vi "2039_hw InitDTTalons.vi"(6 "Brake / Coast Mode":T6, 7 "Ramp Rate (Percent/s)":dbl, 8 "error in (no error)":errorcluster, 10 "Enable VComp":bool, 11 "DT Talon Ref Array":T1[](array[typedef])) -> (0 "error out":errorcluster, 3 "DT Talon Ref Array":T1[](array[typedef]))   [LabVIEW 2016, in "2039lib.lvlib"]
uses:
  2039lib.lvlib
  <vilib>/Rock Robotics/WPI/MotorControl/WPI_MotorControlDeviceRef.ctl
  <vilib>/Rock Robotics/WPI/MotorControl/WPI_MotorControlType.ctl
  <vilib>/Rock Robotics/SystemInterfaces/DIO/FPGA_DIOPWMChannel.ctl
  <vilib>/Rock Robotics/WPI/PWM/WPI_PWMDeadband.ctl
  <vilib>/Rock Robotics/WPI/ThirdParty/CanMotor/TalonSRX/WPI_CANTalonSRX_BrakeOverride.ctl
  <vilib>/Rock Robotics/WPI/ThirdParty/CanMotor/TalonSRX/WPI_CANTalonSRX_APIFeedbackSelect.ctl
  <vilib>/Rock Robotics/WPI/ThirdParty/CanMotor/TalonSRX/WPI_CANTalonSRX_APIControlMode.ctl
panel:
  in  "Feedback Reference":T5
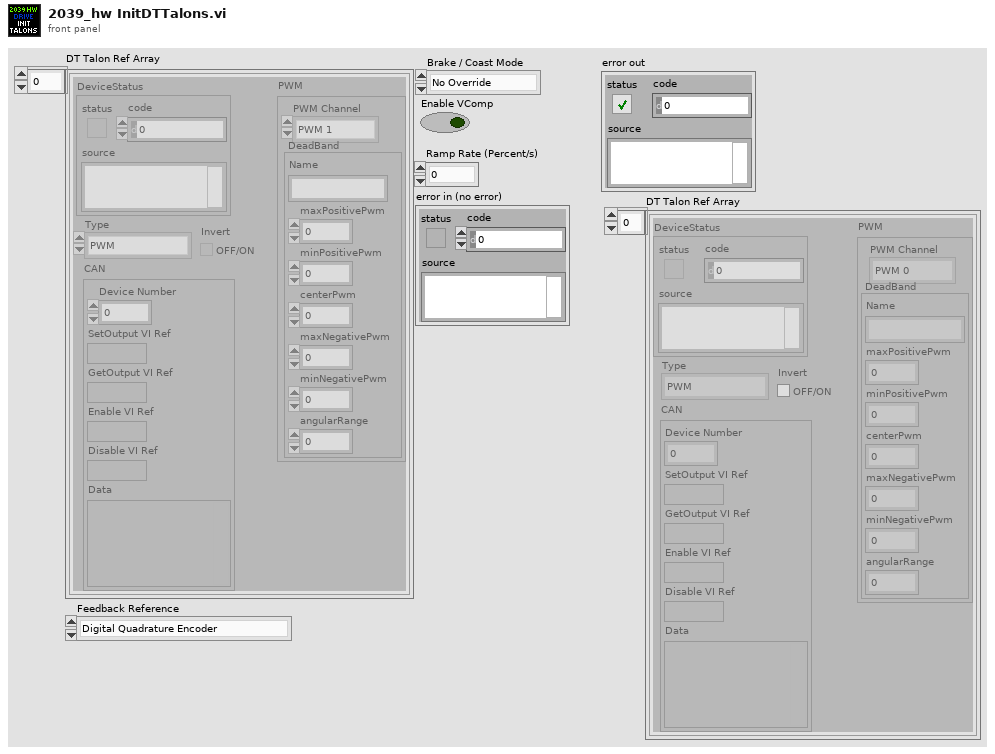
[diagram p1: front panel]
types:
  T1 = typedef "WPI_MotorControlDeviceRef.ctl" = cluster{"DeviceStatus":errorcluster, "Type":T2, "PWM":cluster{"PWM Channel":T3, "DeadBand":T4}, "CAN":cluster{"Device Number":u8, "SetOutput VI Ref":variant, "GetOutput VI Ref":variant, "Enable VI Ref":variant, "Disable VI Ref":variant, "Data":variant}, "Invert":bool}
  T2 = typedef "WPI_MotorControlType.ctl" = enum16{"PWM", "CAN"}
  T3 = typedef "FPGA_DIOPWMChannel.ctl" = enum8{"PWM 0", "PWM 1", "PWM 2", "PWM 3", "PWM 4", "PWM 5", "PWM 6", "PWM 7", "PWM 8", "PWM 9", "PWM MXP 0", "PWM MXP 1", "PWM MXP 2", "PWM MXP 3", "PWM MXP 4", "PWM MXP 5", "PWM MXP 6", "PWM MXP 7", "PWM MXP 8", "PWM MXP 9", "Invalid"}
  T4 = typedef "WPI_PWMDeadband.ctl" = cluster{"Name":string, "maxPositivePwm":i32, "minPositivePwm":i32, "centerPwm":i32, "maxNegativePwm":i32, "minNegativePwm":i32, "angularRange":u16}
  T5 = typedef "WPI_CANTalonSRX_APIFeedbackSelect.ctl" = enum16{"Digital Quadrature Encoder", "Analog Potentiometer", "Analog Encoder", "Count on Quad-A (Rising-Edge)", "Count on Quad-A (Falling-Edge)", "CTR Magnetic Enc (Absolute)", "CTR Magnetic Enc (Relative)", "Pulse Width"}
  T6 = typedef "WPI_CANTalonSRX_BrakeOverride.ctl" = enum8{"No Override", "Override to Coast", "Override to Brake"}
  T7 = typedef "WPI_CANTalonSRX_APIControlMode.ctl" = enum8{"Percent VBus", "Speed", "Position", "Slave", "Unchanged / Invalid", "Voltage Compensation", "Current", "Motion Profile", "Motion Magic"}
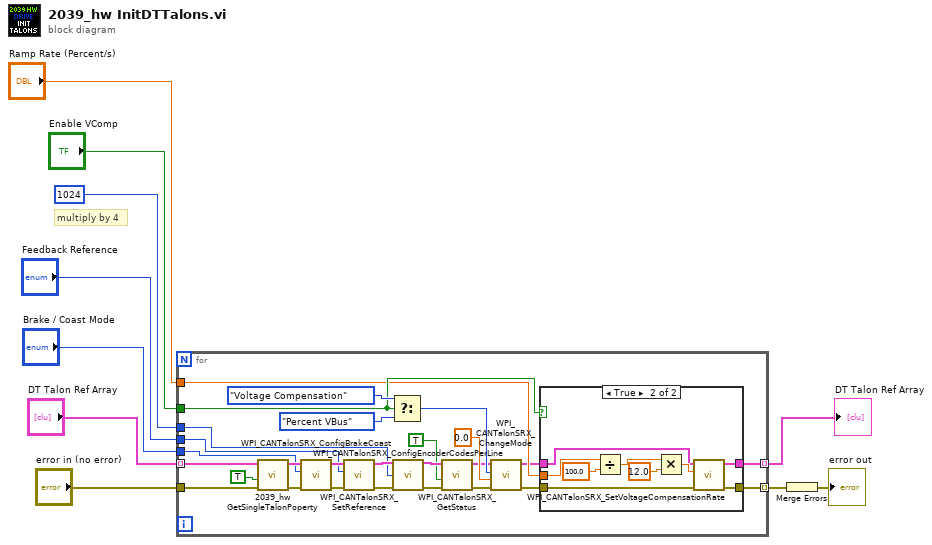
[diagram p0: block diagram]
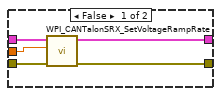
[diagram p2: hidden frame]
diagram:
  # "multiply by 4"
  n1 = for {
    tunnel: "DT Talon Ref Array" -> [w37] mode=indexing
    tunnel: "Brake / Coast Mode" -> [w33]
    tunnel: "Feedback Reference" -> [w30]
    tunnel: "Enable VComp" -> [w25]
    tunnel: "Ramp Rate (Percent/s)" -> [w24]
    tunnel: [w21] -> w2 mode=indexing
    tunnel: [w20] -> w5 mode=indexing
    tunnel: "error in (no error)" -> [w19]
    tunnel: u32 1024 ("Number Encoder Lines\n(Counts Per Rotation)") -> [w17]
    n2 = call "2039_hw GetSingleTalonPoperty.vi"("error in (no error)"=w19, "Clear Sticky Faults"=TRUE, "CAN Talon SRX Ref"=w37) -> ("error out"=w35:errorcluster, "CAN Talon SRX Ref"=w34:T1)  [unwired: 6 in, 1 out]
    n3 = call <vilib>:"WPI_CANTalonSRX_ConfigBrakeCoast.vi"("error in (no error)"=w35, "Brake / Coast Mode"=w33, "CAN Talon SRX Ref"=w34) -> ("error out"=w32:errorcluster, "CAN Talon SRX Ref"=w31:T1)  [unwired: 7 in]
    n4 = call <vilib>:"WPI_CANTalonSRX_SetReference.vi"("error in (no error)"=w32, "Feedback Reference"=w30, "CAN Talon SRX Ref"=w31) -> ("error out"=w14:errorcluster, "CAN Talon SRX Ref"=w18:T1)  [unwired: 7 in]
    n5 = Select(t=WPI_CANTalonSRX_APIControlMode."Voltage Compensation" ("Control Mode"), s=w25, f=WPI_CANTalonSRX_APIControlMode."Percent VBus" ("Control Mode")) -> (s? t:f=w26:T7)
    n6 = call <vilib>:"WPI_CANTalonSRX_ConfigEncoderCodesPerLine.vi"("CAN Talon SRX Ref"=w18, "Number Encoder Lines\n(Counts Per Rotation)"=w17, "error in (no error)"=w14) -> ("CAN Talon SRX Ref"=w15:T1, "error out"=w16:errorcluster)  [unwired: 11 in]
    n7 = call <vilib>:"WPI_CANTalonSRX_GetStatus.vi"("error in (no error)"=w16, "Clear Sticky Faults"=TRUE, "CAN Talon SRX Ref"=w15) -> ("error out"=w11:errorcluster, "CAN Talon SRX Ref"=w13:T1)  [unwired: 6 in, 1 out]
    n8 = call <vilib>:"WPI_CANTalonSRX_ChangeMode.vi"("error in (no error)"=w11, "Output"=0.0, "Control Mode"=w26, "CAN Talon SRX Ref"=w13) -> ("error out"=w22:errorcluster, "CAN Talon SRX Ref"=w23:T1)  [unwired: 6 in]
    n9 = case shown="True" w25 {
      tunnel: w24 -> [w42 w51]
      tunnel: w23 -> [w41 w46]
      tunnel: w22 -> [w40 w45]
      tunnel: [w38 w44] -> w21
      tunnel: [w39 w43] -> w20
      frame False {
        n10 = call <vilib>:"WPI_CANTalonSRX_SetVoltageRampRate.vi"("error in (no error)"=w40, "Throttle Ramp Rate (percent/s)"=w42, "CAN Talon SRX Ref"=w41) -> ("error out"=w39:errorcluster, "CAN Talon SRX Ref"=w38:T1)  [unwired: 7 in]
      }
      frame True {
        n11 = Divide(x=w51, y=100.0) -> (x/y=w49:dbl)
        n12 = Multiply(x=w49, y=12.0) -> (x*y=w47:dbl)
        n13 = call <vilib>:"WPI_CANTalonSRX_SetVoltageCompensationRate.vi"("error in (no error)"=w45, "Voltage Compensation Rate(V/s)"=w47, "CAN Talon SRX Ref"=w46) -> ("error out"=w43:errorcluster, "CAN Talon SRX Ref"=w44:T1)  [unwired: 7 in]
      }
    }
  }
  "DT Talon Ref Array" <- w2
  n14 = Merge Errors(w5) -> (→"error out":errorcluster)
